vi "dfd_FLP IIR I.vi"(7 "x":dbl format="%.2f", 8 "y states in":dbl[](array[numeric]) format="%.2f", 9 "x states in":dbl[](array[numeric]) format="%.2f", 10 "coefficients a":dbl[](array[numeric]) format="%.2f", 11 "coefficents b":dbl[](array[numeric]) format="%.2f") -> (0 "y states out":dbl[](array[numeric]) format="%.2f", 1 "x states out":dbl[](array[numeric]) format="%.2f", 3 "y":dbl format="%.2f")   [LabVIEW 2017, in "NI_DigFilter_FXP.lvlib"]
uses:
  <vilib>/addons/Digital Filter Design/NI_DigFilter_FXP.lvlib
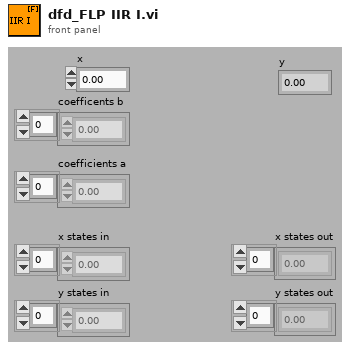
[diagram p1: front panel]
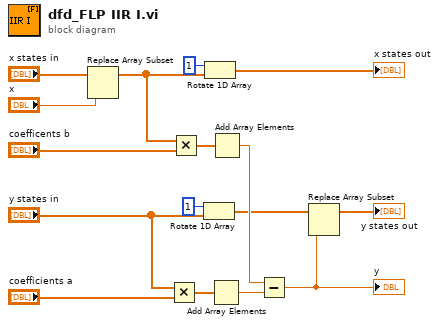
[diagram p0: block diagram]
diagram:
  n1 = Replace Array Subset(array="x states in", new element="x") -> (w10:dbl[])  [unwired: 1 in]
  n2 = Multiply(x="y states in", y="coefficients a") -> (x*y=w12:dbl[])
  n3 = Multiply(x=w10, y="coefficents b") -> (x*y=w14:dbl[])
  n4 = Rotate 1D Array(1:"y states in", 2:1 ("n")) -> (0:w3:dbl[])
  n5 = Rotate 1D Array(1:w10, 2:1 ("n")) -> (0:→"x states out":dbl[])
  n6 = Add Array Elements(numeric array=w12) -> (sum=w15:dbl)
  n7 = Add Array Elements(numeric array=w14) -> (sum=w13:dbl)
  n8 = Subtract(x=w13, y=w15) -> (x-y=w2:dbl)
  "y" <- w2
  n9 = Replace Array Subset(array=w3, new element=w2) -> (→"y states out":dbl[])  [unwired: 1 in]
